vi "send_trigger.vi"(8 "error in (no error)":errorcluster, 10 "trigger":T1, 11 "GenericDisplay in":refnum<class "GenericDisplay.lvclass">) -> (0 "error out":errorcluster, 3 "GenericDisplay out":refnum<class "GenericDisplay.lvclass">)   [LabVIEW 2010, in "GenericDisplay.lvclass"]
uses:
  GenericDisplay.lvclass
  trigger_enum.ctl
  common/classes/GenericToplevelComponent/GenericToplevelComponent/trigger_type_enum.ctl
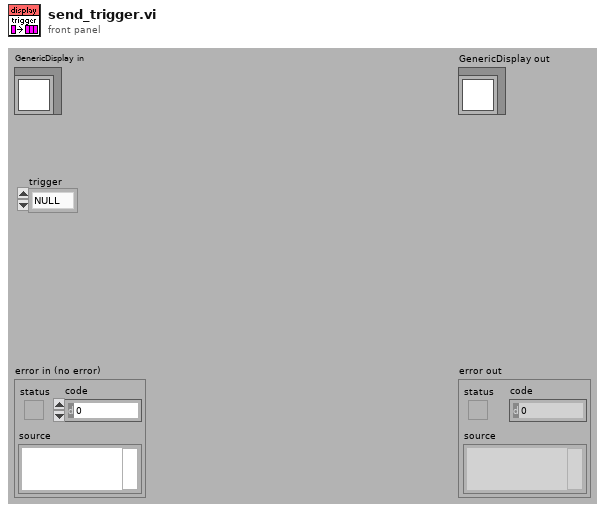
[diagram p1: front panel]
types:
  T1 = typedef "GenericDisplay.lvclass/trigger_enum.ctl" = enum8{"NULL", "display"}
  T2 = typedef "trigger_type_enum.ctl" = enum8{"external", "internal", "common"}
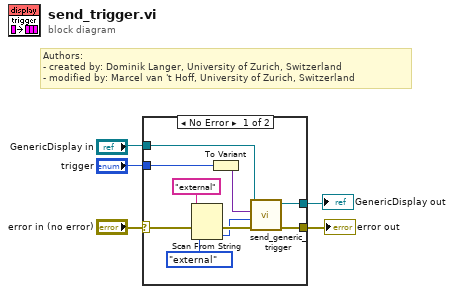
[diagram p0: block diagram]
diagram:
  # "Authors: \n- created by: Dominik Langer, University of Zurich, Switzerland\n- modified by: Marcel van 't Hoff, University of Zurich, Switzerland"
  n1 = case shown="No Error" "error in (no error)" {
    selector: "error in (no error)" -> [w8 w17]
    tunnel: [w15 w17] -> w1
    tunnel: [w12 w16] -> w3
    tunnel: "GenericDisplay in" -> [w11 w16]
    tunnel: "trigger" -> [w14 _]
    frame No Error {
      n2 = Scan From String(input string="external", error in=w8, default 1=trigger_type_enum."external" ("trigger type")) -> (error out=w7:errorcluster, output 1=w6:T2)  [unwired: 2 in, 2 out]
      n3 = To Variant(anything=w14) -> (Variant=w13:variant)
      n4 = call-dynamic "send_generic_trigger.vi"("error in (no error)"=w7, "trigger type"=w6, "trigger variant"=w13, "GenericToplevelComponent in"=w11) -> ("error out"=w15:errorcluster, "GenericToplevelComponent out"=w12:refnum<class "GenericDisplay.lvclass">)  [unwired: 4 in, 2 out]
    }
    frame Error {
    }
  }
  "error out" <- w1
  "GenericDisplay out" <- w3
